vi "MGCC_FntStaMach_Initial_enable.vi"() -> ()   [LabVIEW 2016]
panel:
  out "Data loaded":bool
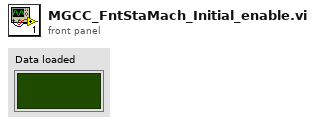
[diagram p1: front panel]
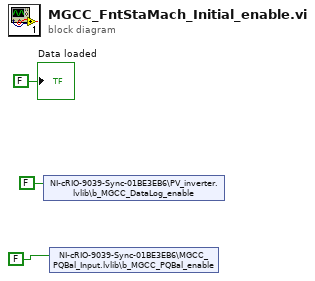
[diagram p0: block diagram]
diagram:
  n1 = shared-variable "NI-cRIO-9039-Sync-01BE3EB6\\PV_inverter.lvlib\\b_MGCC_DataLog_enable"(FALSE ("b_MGCC_DataLog_enable")) -> ()  [unwired: 1 in, 1 out]
  n2 = shared-variable "NI-cRIO-9039-Sync-01BE3EB6\\MGCC_PQBal_Input.lvlib\\b_MGCC_PQBal_enable"(FALSE ("b_MGCC_DataLog_enable")) -> ()  [unwired: 1 in, 1 out]
  "Data loaded" <- FALSE ("Data loaded")
